vi "APC_9049_MFB.vi"(1 "Q":dbl[](array[numeric])) -> (0 "MFB":dbl[](array[numeric]))   [LabVIEW 2020]
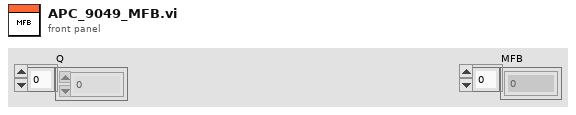
[diagram p1: front panel]
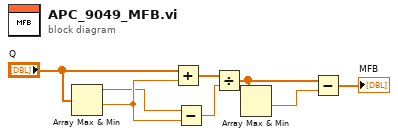
[diagram p0: block diagram]
diagram:
  n1 = Array Max & Min(array="Q") -> (max value=w3:dbl, min value=w4:dbl)  [unwired: 2 out]
  n2 = Add(x="Q", y=w4) -> (x+y=w5:dbl[])
  n3 = Subtract(x=w3, y=w4) -> (x-y=w6:dbl)
  n4 = Divide(x=w5, y=w6) -> (x/y=w8:dbl[])
  n5 = Array Max & Min(array=w8) -> (min value=w7:dbl)  [unwired: 3 out]
  n6 = Subtract(x=w8, y=w7) -> (x-y=→"MFB":dbl[])
